vi "Is Calling VI Running.vi"(8 "Error In":errorcluster, 11 "Calling VI Name":string) -> (0 "Error Out":errorcluster, 3 "Running?":bool)   [LabVIEW 2021, in "Notebook.lvlib"]
uses:
  Notebook.lvlib
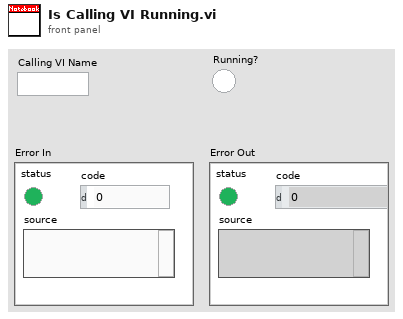
[diagram p1: front panel]
types:
  T1 = enum32{"Bad", "Idle", "Run top level", "Running"}[]
  T2 = enum32{"Invalid", "Standard", "Closed", "Hidden", "Minimized", "Maximized"}[]
  T3 = enum32{"Invalid", "Standard", "Closed", "Hidden", "Minimized", "Maximized"}
  T4 = enum32{"Bad", "Idle", "Run top level", "Running"}
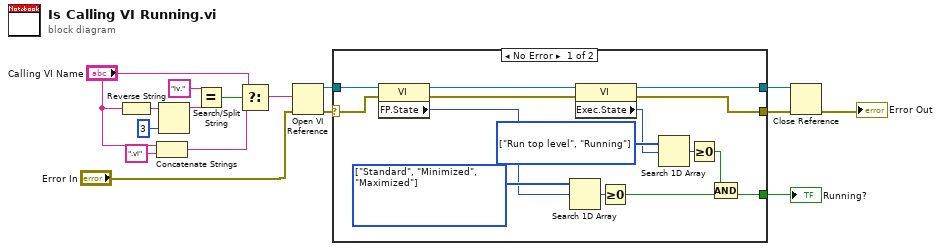
[diagram p0: block diagram]
diagram:
  n1 = Reverse String(1:"Calling VI Name") -> (0:w16:string)
  n2 = Concatenate Strings("Calling VI Name", ".vi" ("string")) -> (w9:string)
  n3 = Search/Split String(string=w16, offset (0)=3) -> (substring before match=w14:string)  [unwired: 1 in, 2 out]
  n4 = Equal?(x="iv.", y=w14) -> (x = y?=w12:bool)
  n5 = Select(t="Calling VI Name", s=w12, f=w9) -> (s? t:f=w3:string)
  n6 = Open VI Reference(vi path=w3, error in (no error)="Error In") -> (vi reference=w8:refnum<vi>, error out=w6:errorcluster)  [unwired: 4 in]
  n7 = case shown="No Error" w6 {
    selector: w6 -> [w30 w32]
    tunnel: w8 -> [w31 w33]
    tunnel: [w22 w33] -> w7
    tunnel: [w24 w32] -> w5
    tunnel: [w18 _] -> w1
    frame No Error {
      w20 = T1 [enum."Run top level", enum."Running"] items=["Bad", "Idle", "Run top level", "Running"] ("Execution:State")
      w28 = T2 [enum."Standard", enum."Minimized", enum."Maximized"] items=["Invalid", "Standard", "Closed", "Hidden", "Minimized", "Maximized"] ("Front Panel Window:State")
      n8 = property class="VI"(reference=w31, error in=w30) -> (reference out=w23:refnum<vi>, error out=w29:errorcluster, "FP.State"=w27:T3)
      n9 = Search 1D Array(1D array=w28, element=w27) -> (index of element=w26:i32)  [unwired: 1 in]
      n10 = property class="VI"(reference=w23, error in=w29) -> (reference out=w22:refnum<vi>, error out=w24:errorcluster, "Exec.State"=w19:T4)
      n11 = Greater Or Equal To 0?(x=w26) -> (x >= 0?=w25:bool)
      n12 = Search 1D Array(1D array=w20, element=w19) -> (index of element=w21:i32)  [unwired: 1 in]
      n13 = Greater Or Equal To 0?(x=w21) -> (x >= 0?=w17:bool)
      n14 = Compound Arithmetic op=AND(w17, w25) -> (w18:bool)
    }
    frame Error {
    }
  }
  "Running?" <- w1
  n15 = Close Reference(reference=w7, error in (no error)=w5) -> (error out=→"Error Out":errorcluster)
